vi "Msg Log Joiner 1.0.vi"(1 "Mode":enum16{"Initialize", "Write"}(ring)=enum."Write", 2 "MSG In":string[][](array[string]), 3 "Table Control":refnum<vi>) -> (0 "Table Out":string[][](table))   [LabVIEW 2014]
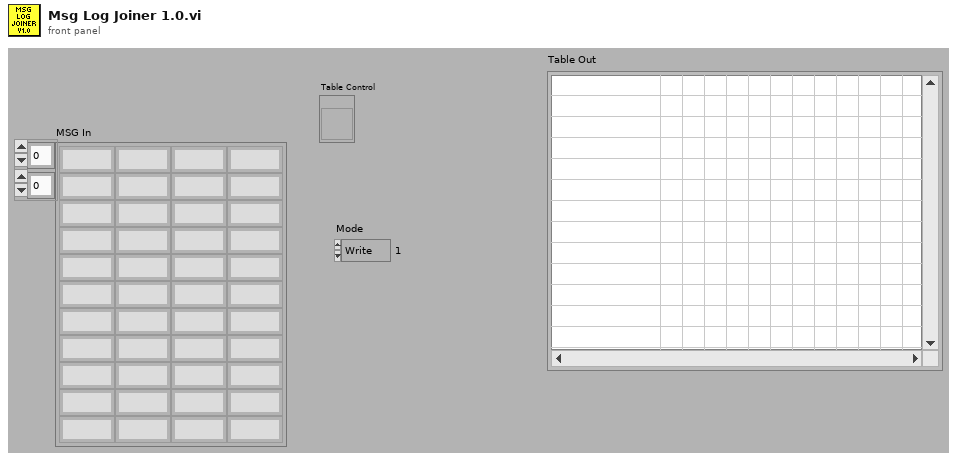
[diagram p1: front panel]
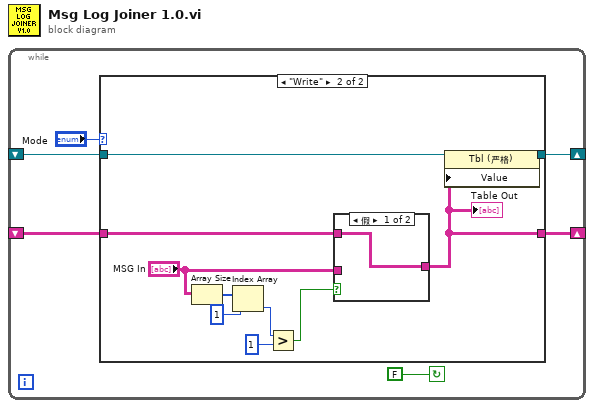
[diagram p0: block diagram]
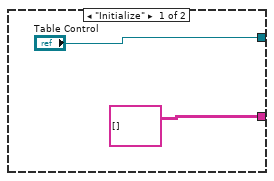
[diagram p2: hidden frame]
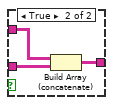
[diagram p3: hidden frame]
diagram:
  n1 = while {
    shift-right: [w4] -> _
    shift-left: _ -> [w3]
    shift-right: [w1] -> _
    shift-left: _ -> [w2]
    stop <- FALSE continue-if-true
    n2 = case shown="\"Write\"" "Mode" {
      tunnel: [string[][] [] w15] -> w4
      tunnel: w3 -> [_ w16]
      tunnel: w2 -> [_ w18]
      tunnel: ["Table Control" w17] -> w1
      frame "Initialize" {
      }
      frame "Write" {
        n3 = Array Size(array="MSG In") -> (size(s)=w13:i32[])
        n4 = Index Array(array=w13, index=1) -> (element=w11:i32)
        n5 = Greater?(x=w11, y=1) -> (0:w12:bool)
        n6 = case shown="假" w12 {
          tunnel: w16 -> [w19 w22]
          tunnel: [w19 w21] -> w15
          tunnel: "MSG In" -> [_ w20]
          frame False {
          }
          frame True {
            n7 = Build Array (concatenate)(w22, w20) -> (w21:string[][])
          }
        }
        "Table Out" <- w15
        n8 = property class="Tbl (严格)"(reference=w18, "Value"=w15) -> (reference out=w17:refnum<vi>)  [unwired: 1 in, 1 out]
      }
    }
  }
